vi "init obj.vi"   [LabVIEW 2017]
doc: "SciScan 1.2 160622"
uses:
  GFG/GFGfpRefGet.vi
  GFG/GFGstringGet.vi
  GFG/GFGnumericGet.vi
  GFG/GFG library.lvlib
types:
  T1 = cluster{"WaveformChartRef":refnum<vi>, "DigitalRef":refnum<vi>, "ArrayRef":refnum<vi>, "TabControlRef":refnum<vi>, "EnumRef":refnum<vi>, "RingRef":refnum<vi>, "BooleanRef":refnum<vi>, "KnobRef":refnum<vi>, "SlideRef":refnum<vi>, "PathRef":refnum<vi>, "StringRef":refnum<vi>, "ComboBox":refnum<vi>, "WaveformGraphRef":refnum<vi>}
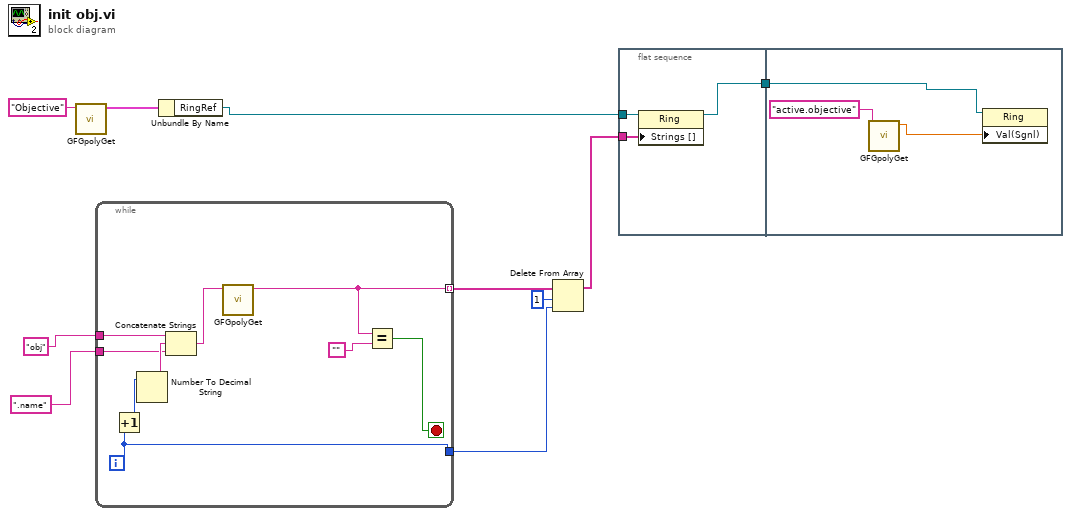
[diagram p0: block diagram]
diagram:
  n1 = call-poly "GFGpolyGet.vi"("Variable Name in"="Objective") -> ("output cluster"=w9:T1)  [unwired: 9 in, 1 out]
  n2 = while {
    tunnel: "obj" ("Variable Name in") -> [w19]
    tunnel: ".name" ("Variable Name in") -> [w16]
    tunnel: [w13] -> w6 mode=indexing
    tunnel: [w11] -> w4
    i -> [w11]
    stop <- w12 stop-if-true
    n3 = Increment(x=w11) -> (x+1=w18:i32)
    n4 = Number To Decimal String(number=w18) -> (decimal integer string=w17:string)  [unwired: 1 in]
    n5 = Concatenate Strings(w19, w17, w16) -> (w15:string)
    n6 = call-poly "GFGpolyGet.vi"("Variable Name in"=w15) -> ("String"=w13:string)  [unwired: 9 in, 1 out]
    n7 = Equal?(x=w13, y="") -> (x = y?=w12:bool)
  }
  n8 = Unbundle By Name(w9) -> ("RingRef"=w3:refnum<vi>)
  n9 = Delete From Array(array=w6, length=1, index=w4) -> (array with subset deleted=w2:string[])  [unwired: 1 out]
  n10 = flat-sequence {
    tunnel: w3 -> [w22]
    tunnel: w2 -> [w21]
    tunnel: [w20] -> w1
    tunnel: w1 -> [w24]
    frame #0 {
      n11 = property class="Ring"(reference=w22, "Strings []"=w21) -> (reference out=w20:refnum<vi>)  [unwired: 1 in, 1 out]
    }
    frame #1 {
      n12 = call-poly "GFGpolyGet.vi"("Variable Name in"="active.objective") -> ("Numeric"=w23:dbl)  [unwired: 8 in, 2 out]
      n13 = property class="Ring"(reference=w24, "Val(Sgnl)"=w23) -> ()  [unwired: 1 in, 2 out]
    }
  }
